vi "Door Booleans.vi"() -> ()   [LabVIEW 2026]
panel:
  in  "Stop":bool
  out "Lock F":bool
  out "Lock E":bool
  out "Lock D":bool
  out "Lock C":bool
  out "Lock B":bool
  out "Lock A":bool
  out "Door F":bool
  out "Door E":bool
  out "Door D":bool
  out "Door C":bool
  out "Door B":bool
  out "Door A":bool
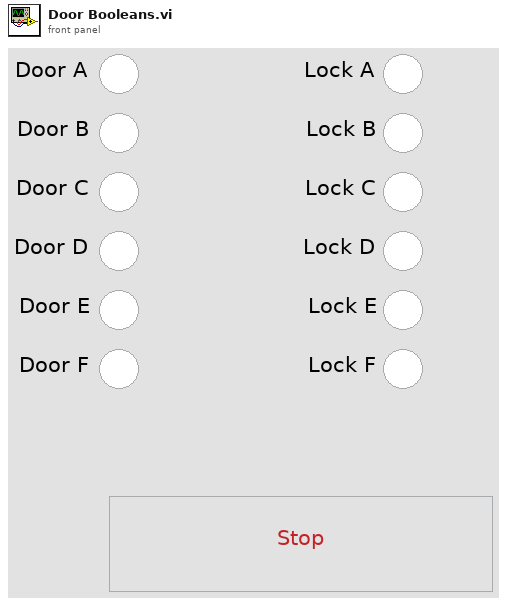
[diagram p1: front panel]
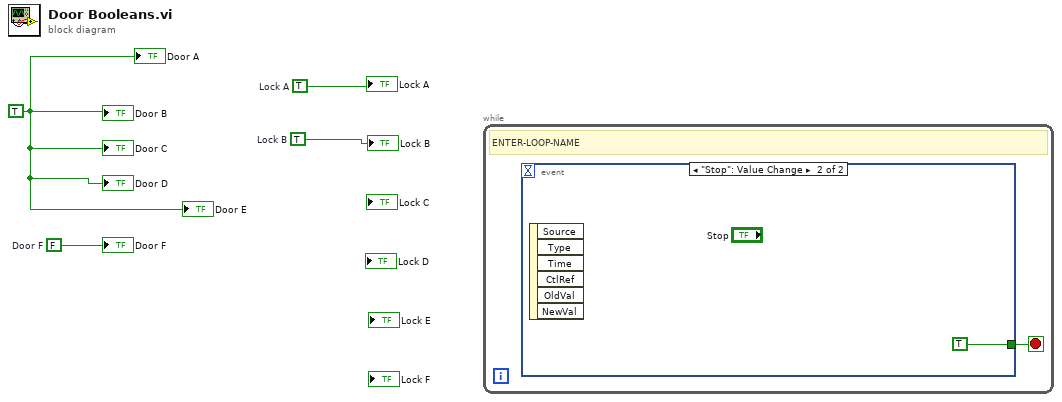
[diagram p0: block diagram]
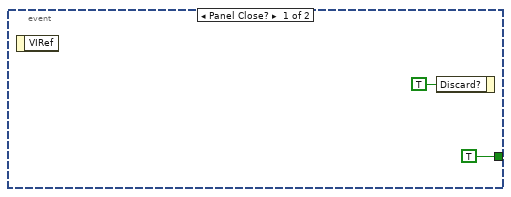
[diagram p2: hidden frame]
diagram:
  w1 = FALSE  # Door F
  w2 = TRUE  # Lock A
  w3 = TRUE  # Lock B
  w4 = TRUE
  n1 = while {
    stop <- w5 stop-if-true
    # "ENTER-LOOP-NAME"
    n2 = event shown="[1] \"Stop\": Value Change" {
      selector: _ -> [_ _]
      dyn-events: _ -> [_ _]
      timeout: _ -> [_ _]
      tunnel: [TRUE TRUE] -> w5
      event Panel Close? {
        n3 = event-data() -> ()  [unwired: 1 in, 1 out]
        n4 = event-data("Discard?"=TRUE) -> ()  [unwired: 1 in, 1 out]
      }
      event "Stop": Value Change {
        n5 = event-data() -> ()  [unwired: 1 in, 6 out]
      }
    }
  }
  "Door A" <- w4
  "Door B" <- w4
  "Door C" <- w4
  "Door D" <- w4
  "Door E" <- w4
  "Door F" <- w1
  "Lock A" <- w2
  "Lock B" <- w3
